vi "Test.vi"() -> ()   [LabVIEW 2013, in "SetUp VIs.lvlib"]
uses:
  SetUp VIs.lvlib
  <instrlib>/Fluke 2625A/Fluke 2625A.lvlib
panel:
  in  "VISA resource name":refnum<visa-resource-name>
  out "read buffer":string
  out "error out":errorcluster
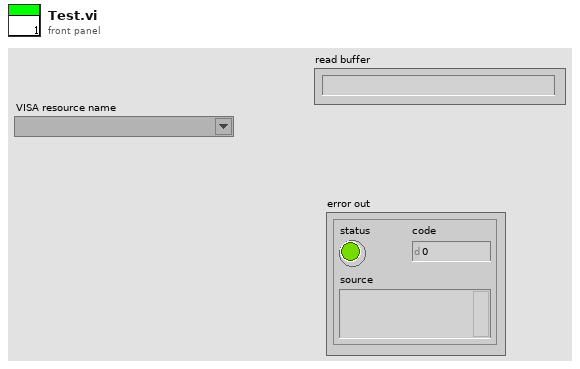
[diagram p1: front panel]
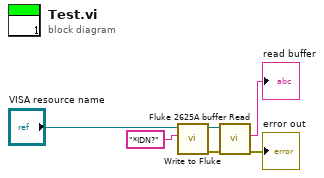
[diagram p0: block diagram]
diagram:
  n1 = call <instrlib>:"Write to Fluke.vi"("write buffer"="*IDN?", "VISA resource name"="VISA resource name") -> ("error out"=w1:errorcluster, "VISA resource name 2"=w3:refnum<visa-resource-name>)  [unwired: 7 in, 1 out]
  n2 = call <instrlib>:"Fluke 2625A buffer Read.vi"("error out"=w1, "VISA resource name out"=w3) -> ("error out 2"=→"error out":errorcluster, "read buffer"=→"read buffer":string)  [unwired: 7 in, 1 out]
